vi "test-units.vi"(8 "error in (no error)":errorcluster) -> (0 "error out":errorcluster, 3 "All Tests Passed":bool)   [LabVIEW 2019]
uses:
  <vilib>/Rock Robotics/WPI/ThirdParty/JAS_Junk/TrajLib/Conv_Deg_Radians.vi
  <vilib>/Rock Robotics/WPI/ThirdParty/JAS_Junk/TrajLib/Conv_Feet_Meters.vi
  <vilib>/Rock Robotics/WPI/ThirdParty/JAS_Junk/TrajLib/Conv_Inches_Meters.vi
  <vilib>/Rock Robotics/WPI/ThirdParty/JAS_Junk/TrajLib/Conv_Meters_Feet.vi
  <vilib>/Rock Robotics/WPI/ThirdParty/JAS_Junk/TrajLib/Conv_Meters_Inches.vi
  <vilib>/Rock Robotics/WPI/ThirdParty/JAS_Junk/TrajLib/Conv_Radians_Deg.vi
  <vilib>/Rock Robotics/WPI/ThirdParty/JAS_Junk/TrajLib/Trajectory_Library.lvlib
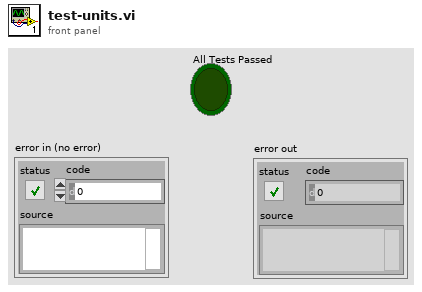
[diagram p1: front panel]
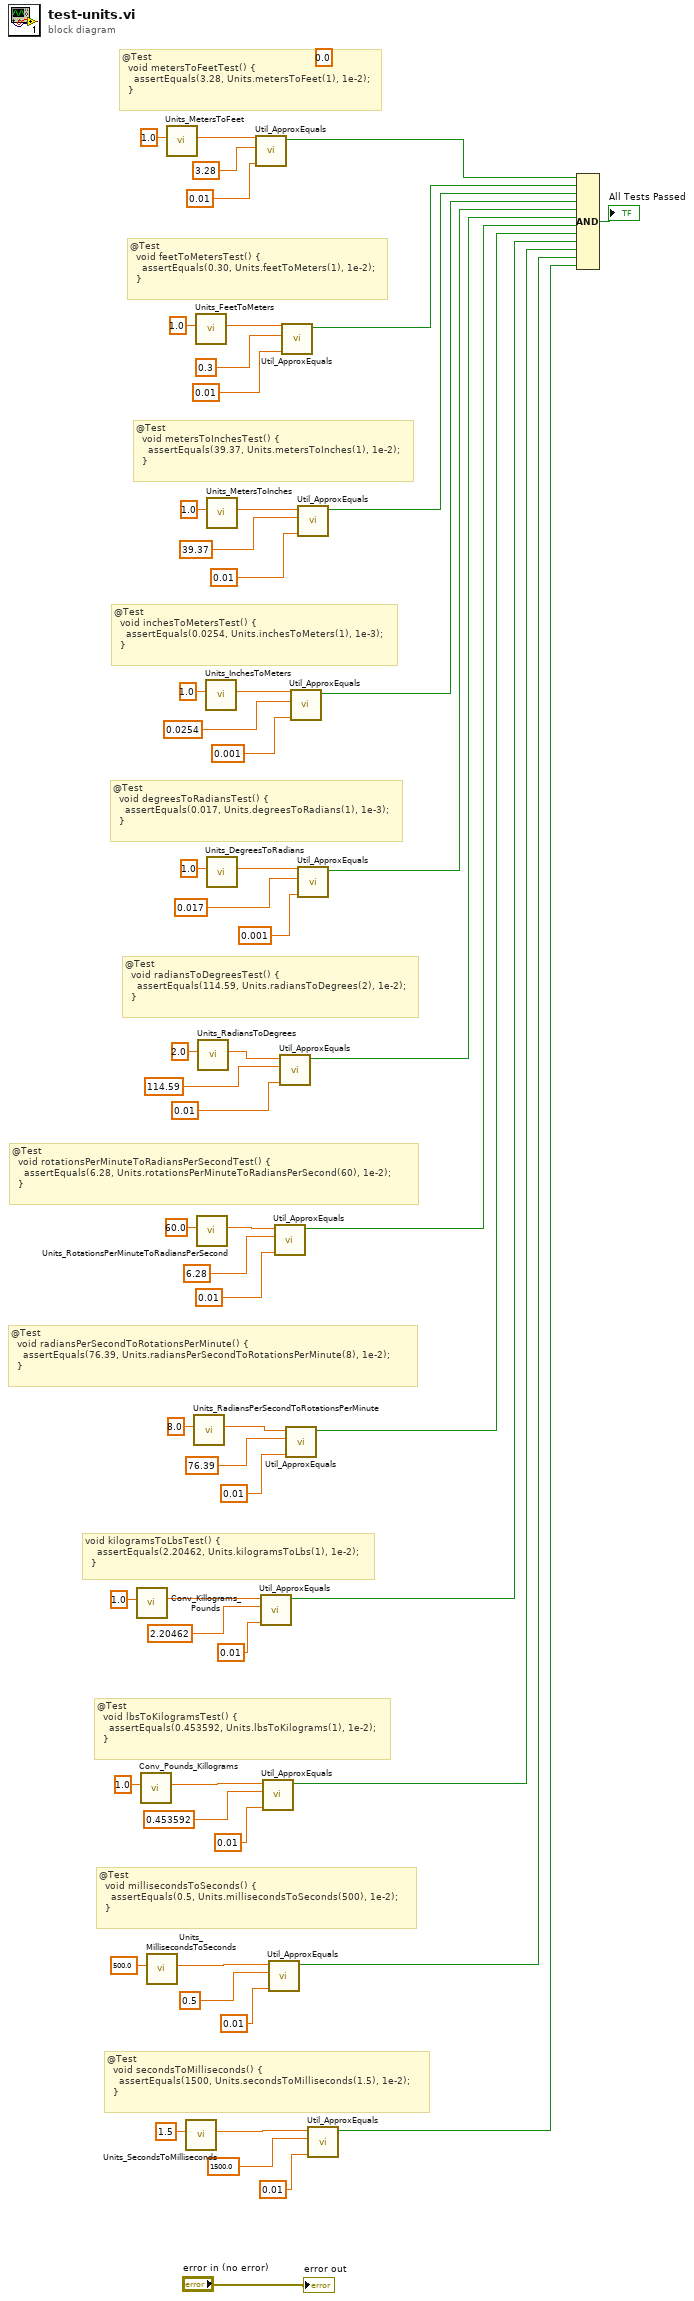
[diagram p0: block diagram]
diagram:
  (unwired) 0.0 ("RotationsPerMinute")
  # "@Test\n  void millisecondsToSeconds() {\n    assertEquals(0.5, Units.millisecondsToSeconds(500), 1e-2);\n  }"
  # "@Test\n  void lbsToKilogramsTest() {\n    assertEquals(0.453592, Units.lbsToKilograms(1), 1e-2);\n  }"
  # "void kilogramsToLbsTest() {\n    assertEquals(2.20462, Units.kilogramsToLbs(1), 1e-2);\n  }"
  # "@Test\n  void radiansPerSecondToRotationsPerMinute() {\n    assertEquals(76.39, Units.radiansPerSecondToRotationsPerMinute(8), 1e-2);\n  }"
  # "@Test\n  void rotationsPerMinuteToRadiansPerSecondTest() {\n    assertEquals(6.28, Units.rotationsPerMinuteToRadiansPerSecond(60), 1e-2);\n  }"
  # "@Test\n  void radiansToDegreesTest() {\n    assertEquals(114.59, Units.radiansToDegrees(2), 1e-2);\n  }"
  # "@Test\n  void degreesToRadiansTest() {\n    assertEquals(0.017, Units.degreesToRadians(1), 1e-3);\n  }"
  # "@Test\n  void inchesToMetersTest() {\n    assertEquals(0.0254, Units.inchesToMeters(1), 1e-3);\n  }"
  # "@Test\n  void metersToInchesTest() {\n    assertEquals(39.37, Units.metersToInches(1), 1e-2);\n  }"
  # "@Test\n  void feetToMetersTest() {\n    assertEquals(0.30, Units.feetToMeters(1), 1e-2);\n  }"
  # "@Test\n  void metersToFeetTest() {\n    assertEquals(3.28, Units.metersToFeet(1), 1e-2);\n  }"
  # "@Test\n  void secondsToMilliseconds() {\n    assertEquals(1500, Units.secondsToMilliseconds(1.5), 1e-2);\n  }"
  n1 = call <vilib>:"Conv_Killograms_Pounds.vi"("Pounds"=1.0) -> ("Killograms"=w21:dbl)  [unwired: 10 in]
  n2 = call <vilib>:"Conv_Pounds_Killograms.vi"("Pounds"=1.0) -> ("Killograms"=w22:dbl)  [unwired: 10 in]
  n3 = call <vilib>:"Units_MillisecondsToSeconds.vi"("Milliseconds"=500.0 ("Pounds")) -> ("Seconds"=w10:dbl)  [unwired: 10 in]
  n4 = call <vilib>:"Units_MetersToFeet.vi"("Meters"=1.0) -> ("Feet"=w55:dbl)  [unwired: 10 in]
  n5 = call <vilib>:"Units_SecondsToMilliseconds.vi"("Seconds"=1.5 ("Pounds")) -> ("Milliseconds"=w6:dbl)  [unwired: 10 in]
  n6 = call <vilib>:"Units_RadiansPerSecondToRotationsPerMinute.vi"("RadiansPerSecond"=8.0) -> ("RotationsPerMinute"=w26:dbl)  [unwired: 10 in]
  n7 = call <vilib>:"Units_FeetToMeters.vi"("Feet"=1.0) -> ("Meters"=w51:dbl)  [unwired: 10 in]
  n8 = call <vilib>:"Units_RotationsPerMinuteToRadiansPerSecond.vi"("RotationsPerMinute"=60.0) -> ("RadiansPerSecond"=w28:dbl)  [unwired: 10 in]
  n9 = call <vilib>:"Units_RadiansToDegrees.vi"("Radians"=2.0) -> ("Degrees"=w36:dbl)  [unwired: 10 in]
  n10 = call <vilib>:"Units_InchesToMeters.vi"("Inches"=1.0) -> ("Meters"=w43:dbl)  [unwired: 10 in]
  n11 = call <vilib>:"Units_MetersToInches.vi"("Meters"=1.0) -> ("Inches"=w47:dbl)  [unwired: 10 in]
  n12 = call <vilib>:"Units_DegreesToRadians.vi"("Degrees"=1.0) -> ("Radians"=w39:dbl)  [unwired: 10 in]
  n13 = call <vilib>:"Util_ApproxEquals.vi"("Tolerance"=0.01, "Value 2"=3.28, "Value 1"=w55) -> ("ApproxEquals"=w52:bool)  [unwired: 8 in]
  n14 = call <vilib>:"Util_ApproxEquals.vi"("Tolerance"=0.01, "Value 2"=2.20462, "Value 1"=w21) -> ("ApproxEquals"=w14:bool)  [unwired: 8 in]
  n15 = call <vilib>:"Util_ApproxEquals.vi"("Tolerance"=0.01, "Value 2"=0.453592, "Value 1"=w22) -> ("ApproxEquals"=w13:bool)  [unwired: 8 in]
  n16 = call <vilib>:"Util_ApproxEquals.vi"("Tolerance"=0.01, "Value 2"=0.5, "Value 1"=w10) -> ("ApproxEquals"=w2:bool)  [unwired: 8 in]
  n17 = call <vilib>:"Util_ApproxEquals.vi"("Tolerance"=0.01, "Value 2"=6.28, "Value 1"=w28) -> ("ApproxEquals"=w27:bool)  [unwired: 8 in]
  n18 = call <vilib>:"Util_ApproxEquals.vi"("Tolerance"=0.01, "Value 2"=114.59, "Value 1"=w36) -> ("ApproxEquals"=w32:bool)  [unwired: 8 in]
  n19 = call <vilib>:"Util_ApproxEquals.vi"("Tolerance"=0.01, "Value 2"=0.3, "Value 1"=w51) -> ("ApproxEquals"=w48:bool)  [unwired: 8 in]
  n20 = call <vilib>:"Util_ApproxEquals.vi"("Tolerance"=0.01, "Value 2"=76.39, "Value 1"=w26) -> ("ApproxEquals"=w23:bool)  [unwired: 8 in]
  n21 = call <vilib>:"Util_ApproxEquals.vi"("Tolerance"=0.001, "Value 2"=0.0254, "Value 1"=w43) -> ("ApproxEquals"=w40:bool)  [unwired: 8 in]
  n22 = call <vilib>:"Util_ApproxEquals.vi"("Tolerance"=0.01, "Value 2"=39.37, "Value 1"=w47) -> ("ApproxEquals"=w44:bool)  [unwired: 8 in]
  n23 = call <vilib>:"Util_ApproxEquals.vi"("Tolerance"=0.001, "Value 2"=0.017, "Value 1"=w39) -> ("ApproxEquals"=w33:bool)  [unwired: 8 in]
  n24 = call <vilib>:"Util_ApproxEquals.vi"("Tolerance"=0.01, "Value 2"=1500.0, "Value 1"=w6) -> ("ApproxEquals"=w1:bool)  [unwired: 8 in]
  n25 = Compound Arithmetic op=AND(w52, w48, w44, w40, w33, w32, w27, w23, w14, w13, w2, w1) -> (→"All Tests Passed":bool)
  "error out" <- "error in (no error)"
